vi "Entry.vi"(8 "error in (no error)":errorcluster, 11 "New State":refnum<class "Receiver Command.lvclass">) -> (0 "error out":errorcluster, 3 "State out":refnum<class "Receiver Command.lvclass">)   [LabVIEW 2013, in "Receiver.lvlib" / "Receive Commands Using State Actors.lvlib" / "Receiver Command.lvclass"]
doc: "This is an abstract method. Override this method to define the behavior when you enter the state."
uses:
  Receiver Command.lvclass
  Command/Command State Actor.lvclass
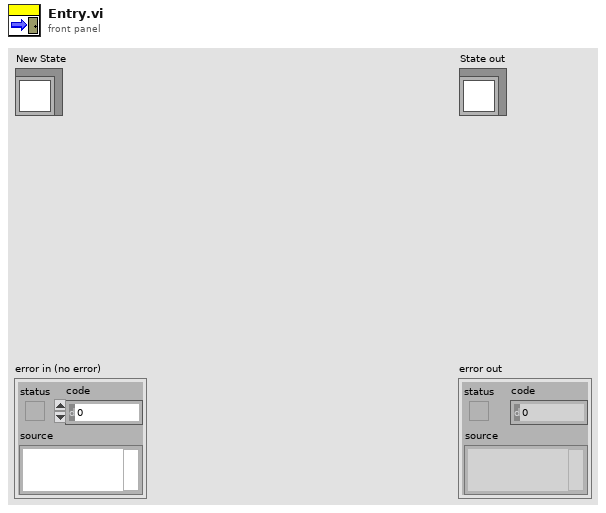
[diagram p1: front panel]
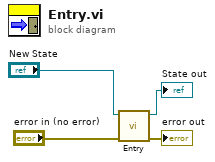
[diagram p0: block diagram]
diagram:
  n1 = call-parent "Entry.vi"("error in (no error)"="error in (no error)", "New State"="New State") -> ("error out"=→"error out":errorcluster, "State out"=→"State out":refnum<class "Receiver Command.lvclass">)  [unwired: 8 in]
